vi "write_params.vi"(8 "error in (no error)":errorcluster, 10 "params":T1={"copy"=TRUE, "fit_intercept"=TRUE, "normalize"=TRUE, "max_iter"={"max_iter_type"="None", "max_iter_int"=0.0}, "cv"=5.0, "n_jobs"=1.0, "verbose"={"verbose_type"="bool", "verbose_bool"=FALSE, "verbose_int"=0.0}}, 11 "OrthogonalMatchingPursuitCV in":refnum<class "OrthogonalMatchingPursuitCV.lvclass">) -> (0 "error out":errorcluster, 3 "OrthogonalMatchingPursuitCV out":refnum<class "OrthogonalMatchingPursuitCV.lvclass">)   [LabVIEW 2020, in "OrthogonalMatchingPursuitCV.lvclass"]
uses:
  OrthogonalMatchingPursuitCV.lvclass
  Controls/orthogonal_matching_pursuit_cv_params.ctl
  OrthogonalMatchingPursuitCV.lvclass/OrthogonalMatchingPursuitCV.ctl
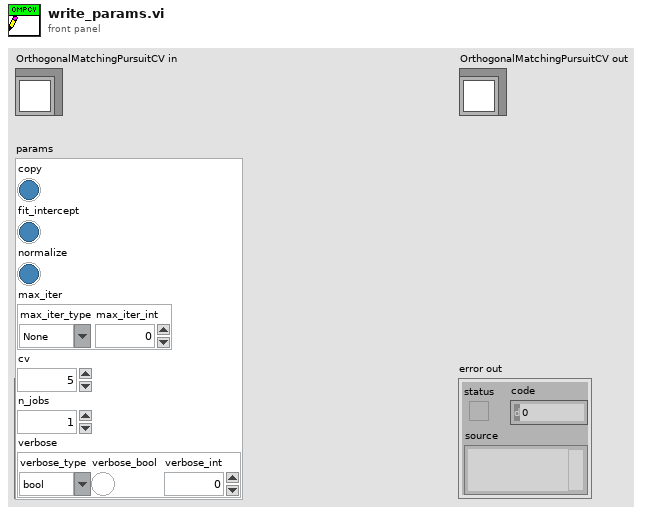
[diagram p1: front panel]
types:
  T1 = typedef "orthogonal_matching_pursuit_cv_params.ctl" = cluster{"copy":bool, "fit_intercept":bool, "normalize":bool, "max_iter":cluster{"max_iter_type":string, "max_iter_int":dbl}, "cv":dbl, "n_jobs":dbl, "verbose":cluster{"verbose_type":string, "verbose_bool":bool, "verbose_int":dbl}}
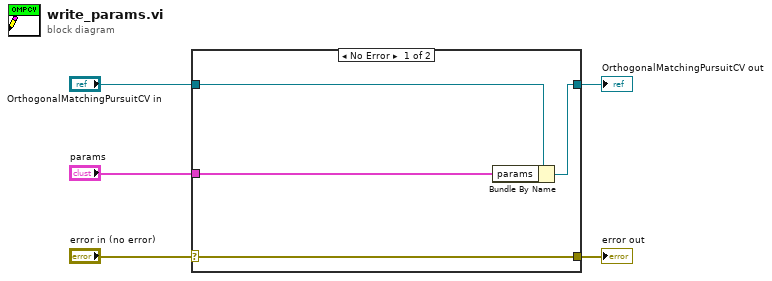
[diagram p0: block diagram]
diagram:
  n1 = case shown="No Error" "error in (no error)" {
    selector: "error in (no error)" -> [w9 w10]
    tunnel: [w9 w10] -> w4
    tunnel: [w7 w11] -> w2
    tunnel: "OrthogonalMatchingPursuitCV in" -> [w8 w11]
    tunnel: "params" -> [w6 _]
    frame No Error {
      n2 = Bundle By Name(cluster=w8, "params"=w6) -> (w7:refnum<class "OrthogonalMatchingPursuitCV.lvclass">)
    }
    frame Error {
    }
  }
  "error out" <- w4
  "OrthogonalMatchingPursuitCV out" <- w2
